vi "Blackbox Data.vi"() -> ()   [LabVIEW 2012]
uses:
  <vilib>/platform/TimedLoop/XDataNode/XDataNode.xnode
  <vilib>/Platform/TimedLoop/XDataNode/nitl_modes.ctl
  <vilib>/Platform/TimedLoop/XDataNode/XDNodeRunTimeDep.lvlib
  <vilib>/Platform/TimedLoop/XDataNode/wakeup.ctl
  <vilib>/Platform/TimedLoop/XDataNode/timing_clust.ctl
  <instrlib>/Hokuyo URG Series/Hokuyo URG Series.lvlib
  <instrlib>/Hokuyo URG Series/Public/Initialize-Standard.vi
panel:
  in  "VISA resource name":refnum<visa-resource-name>
  out "error out":errorcluster
  in  "stop?":bool
  in  "start point (-135°)":dbl=-135.0
  in  "end point (135°)":dbl=135.0
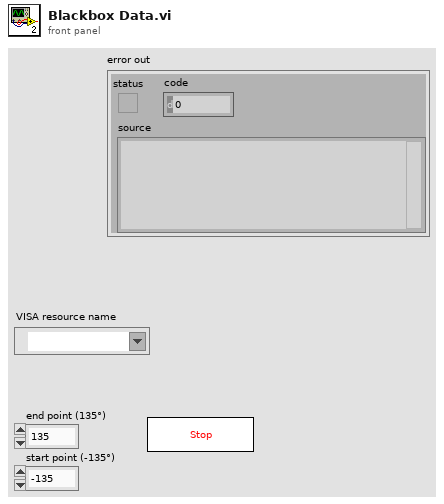
[diagram p1: front panel]
types:
  T1 = enum16{"open", "open or create", "create or replace", "create", "open (read-only)"}
  T2 = typedef "XDNodeRunTimeDep.lvlib/timing_clust.ctl" = cluster{"Expected End [f-1]":u64, "Actual End [f-1]":u64, "Finished Late? [f-1]":bool, "Expected End [i-1]":u64, "Actual End [i-1]":u64, "Finished Late? [i-1]":bool, "Expected Start [i]":u64, "Actual Start [i]":u64, "Expected Start [f]":u64, "Actual Start [f]":u64, "Source Name":string, "Structure Name":string, "Period":i64, "Deadline":i64, "Offset":i64, "Start":i64, "Priority":i32, "Timeout":i32, "Mode":T3, "Wakeup Reason":T4, "Error":errorcluster, "Source Type":string, "Secondary Source Type":string, "Global End Time":u64, "Global Start Time":u64, "Frame Duration":u64, "Iteration Duration":u64, "Assigned CPU":i32, "I/O Scan Engine Mode":u32}
  T3 = typedef "XDNodeRunTimeDep.lvlib/nitl_modes.ctl" = enum32{"No Change", "Process missed periods, maintain original phase", "Discard missed periods, maintain original phase", "Process missed periods, ignore original phase", "Discard missed periods, ignore original phase"}
  T4 = typedef "XDNodeRunTimeDep.lvlib/wakeup.ctl" = enum32{"Normal", "Aborted", "Asynchronous wakeup", "Timing source error", "Timed loop error", "Timeout"}
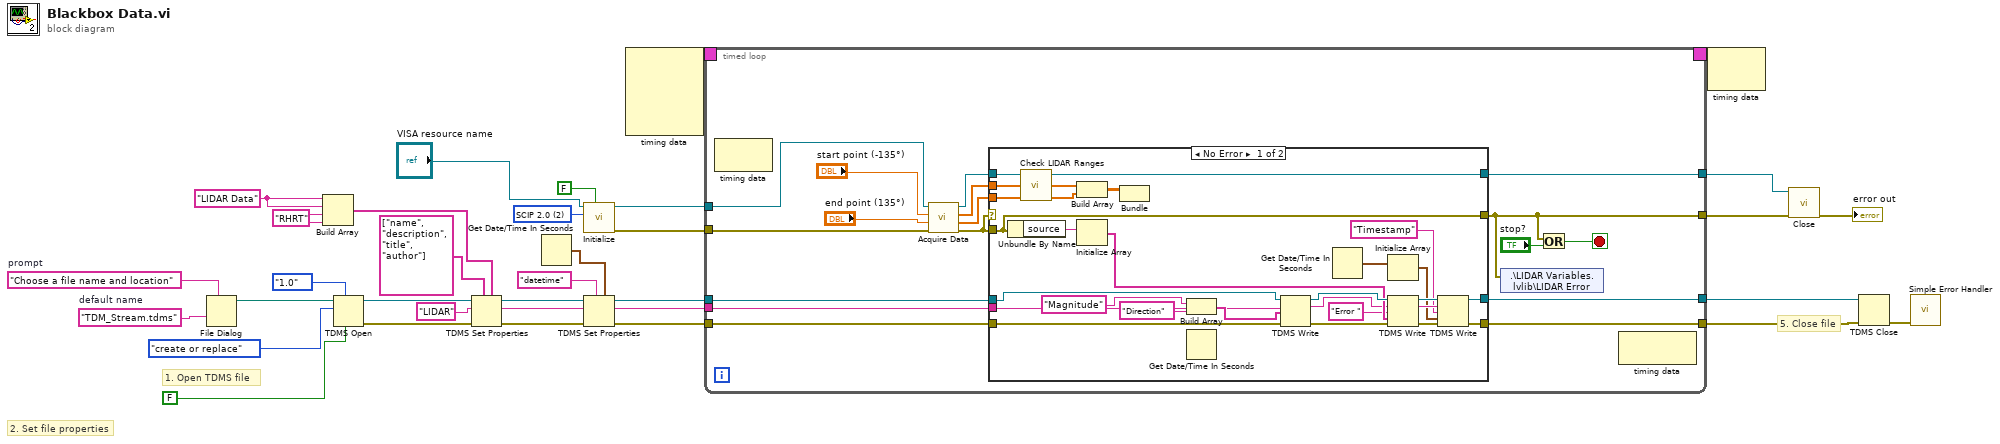
[diagram p0: block diagram]
diagram:
  w5 = u32 2 items=["Convert to Latest", "SCIP 1.1", "SCIP 2.0"] ("Protocol (2: SCIP 2.0)")
  w25 = "TDM_Stream.tdms"  # default name
  w26 = "Choose a file name and location"  # prompt
  w32 = "RHRT" ("title")
  w33 = "LIDAR Data" ("name")
  # "5. Close file"
  # "2. Set file properties"
  # "1. Open TDMS file"
  n1 = File Dialog(7:w26, 9:w25) -> (3:w21:path)  [unwired: 1 in, 7 out]
  n2 = Build Array(w33, w33, w32, w32) -> (w31:string[])
  n3 = TDMS Open(6:FALSE ("disable buffering (T)"), 7:enum16{"1.0", "2.0"}."1.0" ("file format version (2.0)"), 10:T1."create or replace" ("operation"), 11:w21) -> (0:w22:errorcluster, 3:w23:refnum<k34>)  [unwired: 2 in]
  n4 = TDMS Set Properties(5:w31, 7:string[] ["name", "description", "title", "author"] ("property names"), 8:w22, 10:"LIDAR" ("group name in (Untitled)"), 11:w23) -> (0:w30:errorcluster, 2:w2:string, 3:w29:refnum<k34>)  [unwired: 2 out]
  n5 = Get Date/Time In Seconds() -> (seconds since 1Jan1904=w27:timestamp)
  n6 = call-poly <instrlib>:"Initialize.vi"("ID Query? (Enabled)"=FALSE, "Protocol (2: SCIP 2.0)"=w5, "VISA resource name"="VISA resource name") -> ("error out"=w10:errorcluster, "VISA resource name out"=w11:refnum<visa-resource-name>)  [unwired: 7 in]
  n7 = TDMS Set Properties(5:w27, 7:"datetime", 8:w30, 10:w2, 11:w29) -> (0:w8:errorcluster, 2:w1:string, 3:w9:refnum<k34>)  [unwired: 2 out]
  n8 = node-c288() -> (w17:T2)  [unwired: 4 out]
  n9 = timed-loop {
    timing: w17 -> [_]
    timing-out: [_] -> w16
    tunnel: w11 -> [w47]
    tunnel: [w45] -> w15
    tunnel: [w42] -> w14
    tunnel: w10 -> [w43]
    tunnel: w9 -> [w41]
    tunnel: w8 -> [w40]
    tunnel: [w39] -> w7
    tunnel: [w38] -> w6
    tunnel: w1 -> [w35]
    stop <- w36 stop-if-true
    n10 = node-c288() -> ()  [unwired: 2 out]
    n11 = call <instrlib>:"Acquire Data.vi"("error in (no error)"=w43, "End Point (120°)"="end point (135°)", "Start Point (-120°)"="start point (-135°)", "VISA resource name"=w47) -> ("error out"=w44:errorcluster, "Direction"=w50:dbl[], "Magnitude"=w51:dbl[], "VISA resource name out"=w46:refnum<visa-resource-name>)  [unwired: 4 in]
    n12 = case shown="No Error" w44 {
      selector: w44 -> [_ w80]
      tunnel: w51 -> [w76 _]
      tunnel: w50 -> [w68 _]
      tunnel: w46 -> [w77 w81]
      tunnel: [w77 w81] -> w45
      tunnel: [w67 w80] -> w42
      tunnel: w44 -> [w67 _]
      tunnel: w41 -> [w75 w78]
      tunnel: w40 -> [w74 w79]
      tunnel: [w57 w78] -> w39
      tunnel: [w56 w79] -> w38
      tunnel: w35 -> [w52 _]
      frame No Error {
        n13 = Unbundle By Name(w67) -> ("source"=w64:string)
        n14 = call "Check LIDAR Ranges.vi"("Magnitude"=w76) -> ("Magnitude out"=w73:dbl[])  [unwired: 4 in]
        n15 = Build Array(w73, w68) -> (w69:dbl[][])
        n16 = Initialize Array(w64) -> (w63:string[])  [unwired: 1 in]
        n17 = Bundle(w69) -> ()  [unwired: 2 in, 1 out]
        n18 = Build Array("Magnitude", "Direction") -> (w72:string[])
        n19 = Get Date/Time In Seconds() -> ()  [unwired: 1 out]
        n20 = TDMS Write(0:w75, 5:w52, 7:w72, 11:w74) -> (4:w66:refnum<k34>, 6:w62:string, 15:w65:errorcluster)  [unwired: 2 in, 1 out]
        n21 = Get Date/Time In Seconds() -> (seconds since 1Jan1904=w55:timestamp)
        n22 = Initialize Array(w55) -> (w54:timestamp[])  [unwired: 1 in]
        n23 = TDMS Write(0:w66, 5:w62, 7:"Error " ("channel name(s) in (Untitled)"), 9:w63, 11:w65) -> (4:w58:refnum<k34>, 6:w60:string, 15:w59:errorcluster)  [unwired: 1 in, 1 out]
        n24 = TDMS Write(0:w58, 5:w60, 7:"Timestamp" ("channel name(s) in (Untitled)"), 9:w54, 11:w59) -> (4:w57:refnum<k34>, 15:w56:errorcluster)  [unwired: 1 in, 2 out]
      }
      frame Error {
      }
    }
    n25 = shared-variable ".\\LIDAR Variables.lvlib\\LIDAR Error"(w42) -> ()  [unwired: 1 in, 1 out]
    n26 = Or(x=w42, y="stop?") -> (x .or. y?=w36:bool)
    n27 = node-c288() -> ()  [unwired: 2 out]
  }
  n28 = node-c288(w16) -> ()  [unwired: 1 out]
  n29 = call <instrlib>:"Close.vi"("error in (no error)"=w14, "VISA resource name"=w15) -> ("error out"=→"error out":errorcluster)  [unwired: 9 in]
  n30 = TDMS Close(8:w6, 11:w7) -> (0:w20:errorcluster)  [unwired: 1 out]
  n31 = call <vilib>:"Simple Error Handler.vi"("error in (no error)"=w20) -> ()  [unwired: 1 in, 8 out]
